vi "Robot Global Data.vi"() -> ()   [LabVIEW 2011]
doc: "This global VI can contain as many global variables as you need. Place a control on the panel, give it a good name. To read or write to it from a VI, drag the icon to the diagram of that VI. You can also drag from the project. Click on the node to change which global you access. You shouldn't have multiple locations writing to a global or it will cause a race-condition."
uses:
  <vilib>/Rock Robotics/WPI/Camera/WPI_CameraImageSize.ctl
  <vilib>/Rock Robotics/WPI/Joystick/WPI_JoystickButtonState.ctl
  UDP Communication Folder/UDP Dashboard Packet TypeDef.ctl
  <vilib>/Rock Robotics/WPI/DriverStation/WPI_DriverStationRobotMode.ctl
panel:
  in  "Ball State Machine":T1
  in  "Auto Load Balls State":bool
  in  "Feed Balls":bool
  out "Tracking":bool
  in  "Shooter Controls":T2
  out "Layup State":enum16{"Layup Left", "Layup Right", "Off"}(ring)=enum."Off"
  in  "Servo Positions In":cluster{"X":dbl, "Y":dbl}
  out "Autonomous Shooter Distance":dbl
  out "Gyro Angle":dbl(knob) scale=0.0..360.0
  out "Automatic Mode":bool
  in  "Joystick Axis":T3
  in  "Robot Mode":T4
  in  "Turret Info":T5
  out "Shooter Info":T6
  out "UDP Reading":bool
  out "Encoders":cluster{"Average":dbl, "Left":dbl, "Right":dbl}
  out "Solenoids":T7
  out "IR Values":T8
  in  "UDP Dashboard Packet":T9={"Distance"=0.0, "Shooter Control"={"Manual Enabled"=FALSE, "Manual Distance"=0.0, "Power Constant"=0.0, "RPM Constant"=0.0, "Layup Distance"=0.0, "RPM Range"={"Max Percentage"=0.0, "Min Percentage"=0.0}, "Dt In"=0.0}, "Tracking Setpoint"=0.0, "Shooter PID gains"={"proportional gain (Kc)"=0.003, "integral time (Ti, min)"=0.0, "derivative time (Td, min)"=0.0}, "Tracking PID gains"={"proportional gain (Kc)"=0.003, "integral time (Ti, min)"=0.0, "derivative time (Td, min)"=0.0}, "Shooter PID gains 2"={"proportional gain (Kc)"=0.003, "integral time (Ti, min)"=0.0, "derivative time (Td, min)"=0.0}, "Tracking Tolerance"=0.05, "Tracking Limit"=0.7, "Autonomous Ball Collection / Shoot Period"=3.5}
  out "Gamepad Axes":T3
  out "Joystick Buttons":T10
  in  "Allow Fire":bool
  out "Buttons":T10
  in  "LED toggle rate (ms)":u32=20
  in  "image size":T11=enum."320x240"
  in  "Enable Vision":bool
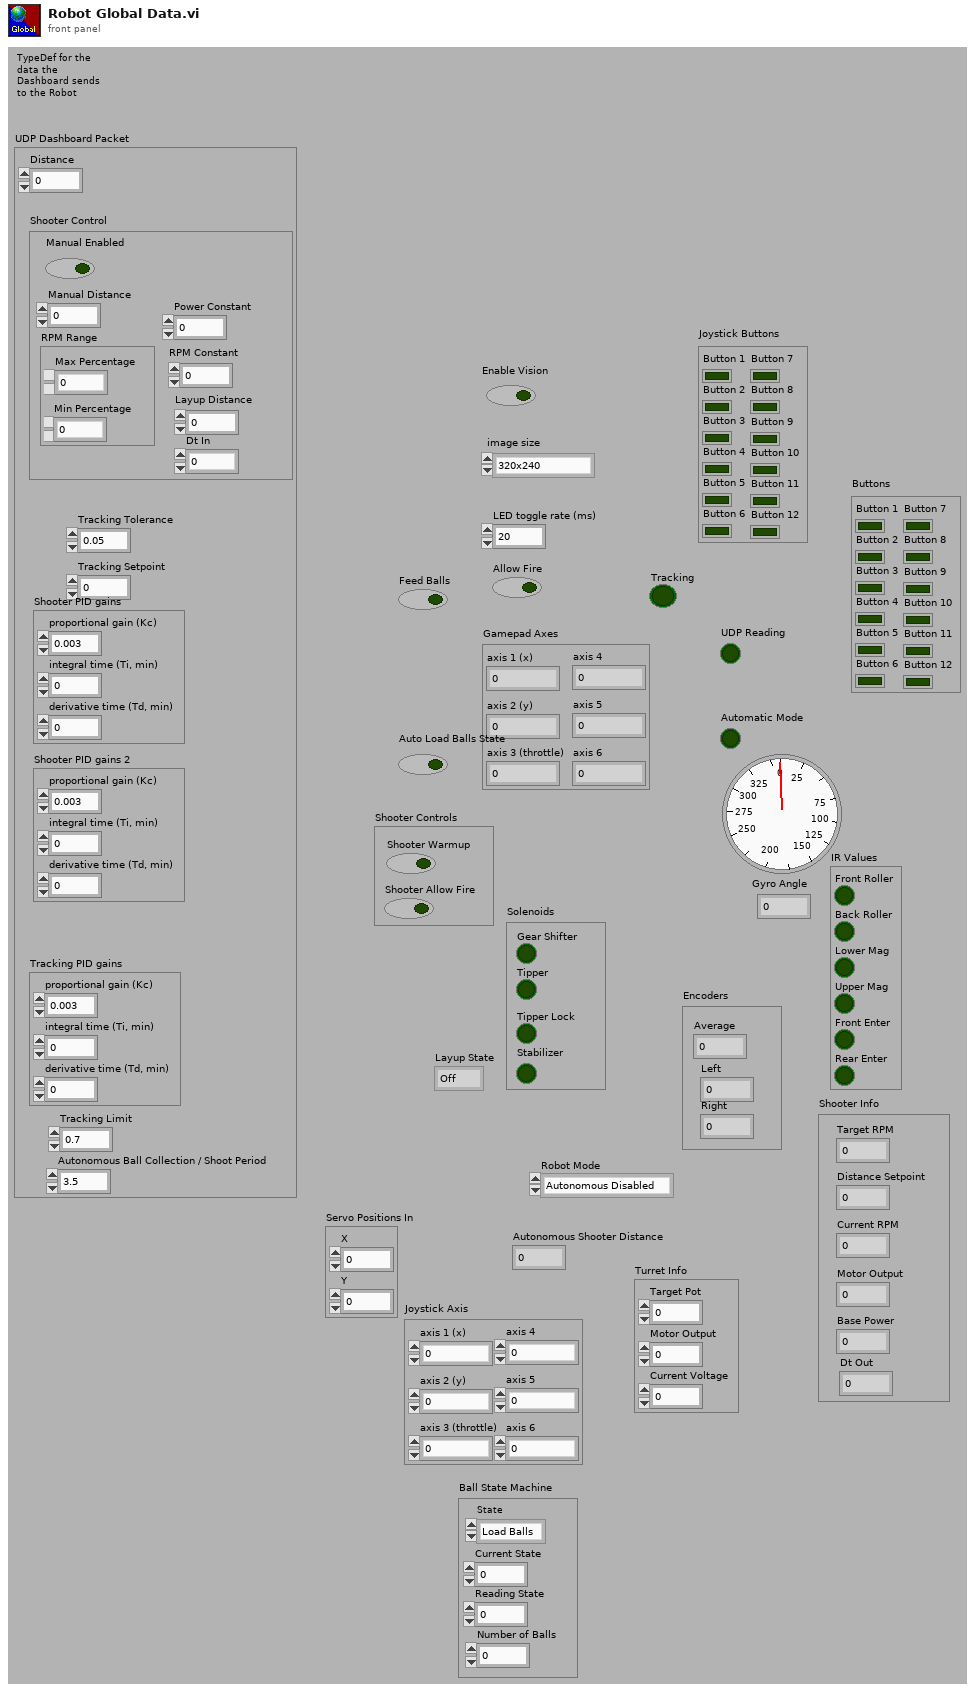
[diagram p1: front panel]
types:
  T1 = cluster{"Current State":u32, "Reading State":u32, "Number of Balls":u32, "State":enum16{"Load Balls", "Shoot", "Wait"}}
  T2 = cluster{"Shooter Warmup":bool, "Shooter Allow Fire":bool}
  T3 = cluster{"axis 1 (x)":dbl, "axis 2 (y)":dbl, "axis 3 (throttle)":dbl, "axis 4":dbl, "axis 5":dbl, "axis 6":dbl}
  T4 = typedef "WPI_DriverStationRobotMode.ctl" = enum16{"Autonomous Disabled", "Autonomous Enabled", "Teleop Disabled", "Teleop Enabled", "Timeout", "Finish"}
  T5 = cluster{"Target Pot":dbl, "Motor Output":dbl, "Current Voltage":dbl}
  T6 = cluster{"Current RPM":dbl, "Distance Setpoint":dbl, "Target RPM":dbl, "Motor Output":dbl, "Base Power":dbl, "Dt Out":dbl}
  T7 = cluster{"Gear Shifter":bool, "Tipper":bool, "Tipper Lock":bool, "Stabilizer":bool}
  T8 = cluster{"Front Roller":bool, "Back Roller":bool, "Lower Mag":bool, "Upper Mag":bool, "Front Enter":bool, "Rear Enter":bool}
  T9 = typedef "UDP Dashboard Packet TypeDef.ctl" = cluster{"Distance":dbl, "Shooter Control":cluster{"Manual Enabled":bool, "Manual Distance":dbl, "Power Constant":dbl, "RPM Constant":dbl, "Layup Distance":dbl, "RPM Range":cluster{"Max Percentage":dbl, "Min Percentage":dbl}, "Dt In":dbl}, "Tracking Setpoint":dbl, "Shooter PID gains":cluster{"proportional gain (Kc)":dbl, "integral time (Ti, min)":dbl, "derivative time (Td, min)":dbl}, "Tracking PID gains":cluster{"proportional gain (Kc)":dbl, "integral time (Ti, min)":dbl, "derivative time (Td, min)":dbl}, "Shooter PID gains 2":cluster{"proportional gain (Kc)":dbl, "integral time (Ti, min)":dbl, "derivative time (Td, min)":dbl}, "Tracking Tolerance":dbl, "Tracking Limit":dbl, "Autonomous Ball Collection / Shoot Period":dbl}
  T10 = typedef "WPI_JoystickButtonState.ctl" = cluster{"Button 1":bool, "Button 2":bool, "Button 3":bool, "Button 4":bool, "Button 5":bool, "Button 6":bool, "Button 7":bool, "Button 8":bool, "Button 9":bool, "Button 10":bool, "Button 11":bool, "Button 12":bool}
  T11 = typedef "WPI_CameraImageSize.ctl" = enum16{"640x480", "320x240", "160x120"}
diagram:
